vi "tragetory generation.vi"(8 "error in":errorcluster, 11 "file path":path) -> (0 "error out":errorcluster, 3 "reference":dbl)   [LabVIEW 2011, in "kevLib2011.lvlib"]
uses:
  kevLib2011.lvlib
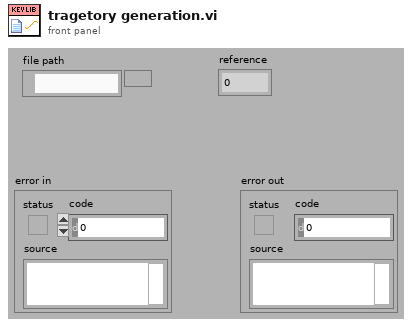
[diagram p1: front panel]
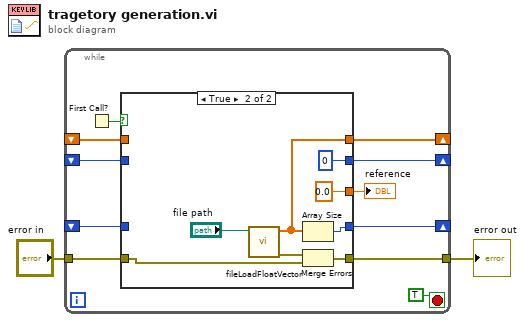
[diagram p0: block diagram]
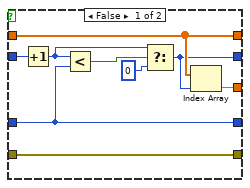
[diagram p2: hidden frame]
diagram:
  n1 = while {
    shift-right: [w10] -> _
    shift-left: _ -> [w8]
    shift-right: [w11] -> _
    shift-left: _ -> [w9]
    shift-right: [w7] -> _
    shift-left: _ -> [w6]
    tunnel: [w4] -> w2
    tunnel: "error in" -> [w3]
    stop <- TRUE stop-if-true
    n2 = First Call?() -> (First Call?: T/F=w13:bool)
    n3 = case shown="True" w13 {
      tunnel: [w21 w27] -> w11
      tunnel: [w18 w26] -> w10
      tunnel: w9 -> [w21 _]
      tunnel: w8 -> [w18 _]
      tunnel: [w17 0 ("f")] -> w7
      tunnel: w6 -> [w20 _]
      tunnel: [w16 0.0 ("Data Type (DBL)")] -> w5
      tunnel: [w14 w23] -> w4
      tunnel: w3 -> [w14 w24]
      frame False {
        n4 = Increment(x=w20) -> (x+1=w15:i32)
        n5 = Less?(x=w15, y=w21) -> (x < y?=w22:bool)
        n6 = Select(t=w15, s=w22, f=0) -> (s? t:f=w17:i32)
        n7 = Index Array(array=w18, index=w17) -> (element=w16:dbl)
      }
      frame True {
        n8 = call "fileLoadFloatVector.vi"("File Path"="file path") -> ("error out"=w25:errorcluster, "Float Vector"=w26:dbl[])  [unwired: 9 in]
        n9 = Array Size(array=w26) -> (size(s)=w27:i32)
        n10 = Merge Errors(w25, w24) -> (w23:errorcluster)
      }
    }
    "reference" <- w5
  }
  "error out" <- w2
